vi "DidStop.vi"(8 "ErrorArray In":errorcluster[](array[cluster]), 10 "Init?":bool, 11 "NISTBus In":refnum<class "NISTBus.lvclass">) -> (0 "ErrorArray Out":errorcluster[](array[cluster]), 3 "NISTBus Out":refnum<class "NISTBus.lvclass">)   [LabVIEW 2014, in "Bus.lvlib"]
uses:
  Bus.lvlib
  NISTBus.lvclass
  Typedefs/clDidInit.ctl
  Typedefs/clUserEventType.ctl
  <userlib>/NIST/NISTErrorLib/NISTErrorLib.lvlib
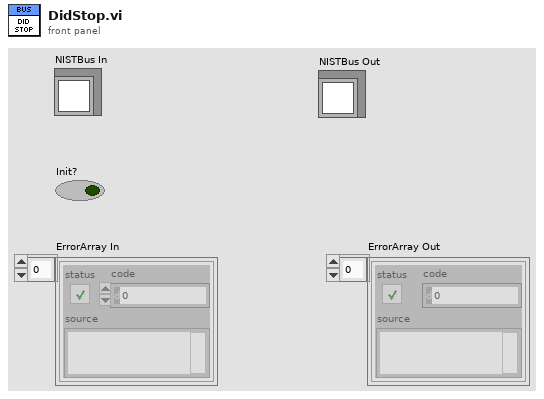
[diagram p1: front panel]
types:
  T1 = typedef "Bus.lvlib/clUserEventType.ctl" = cluster{"BusNumber":i8, "Data":variant}
  T2 = typedef "Bus.lvlib/clDidInit.ctl" = cluster{"NISTBus":refnum<vi>, "Init?":bool}
  T3 = typedef "Bus.lvlib/clBroadcastEvents.ctl" = cluster{"DidInit":refnum<user-event>, "DidStop":refnum<user-event>}
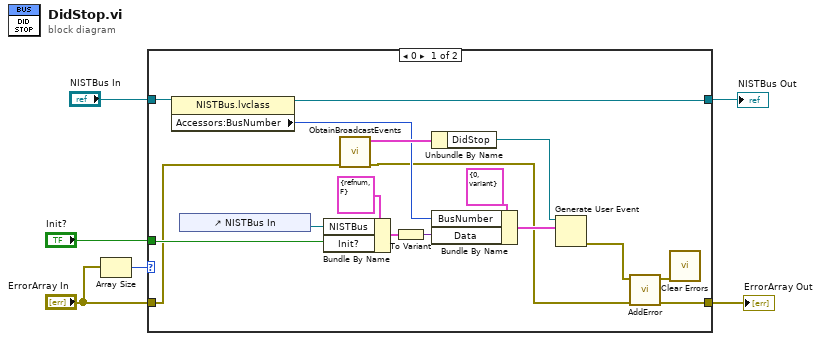
[diagram p0: block diagram]
diagram:
  n1 = Array Size(array="ErrorArray In") -> (size(s)=w6:i32)
  n2 = case shown="0" w6 {
    tunnel: "ErrorArray In" -> [w18 w24]
    tunnel: "Init?" -> [w19 _]
    tunnel: [w22 w25] -> w2
    tunnel: "NISTBus In" -> [w23 w25]
    tunnel: [w9 w24] -> w1
    frame 0 {
      n3 = property class="NISTBus.lvclass"(reference=w23) -> (reference out=w22:refnum<class "NISTBus.lvclass">, "Accessors:BusNumber"=w13:u8)  [unwired: 1 in, 1 out]
      n4 = control-ref of="NISTBus In"() -> (w20:refnum<vi>)
      n5 = Bundle By Name(cluster=T2 {"NISTBus"=refnum, "Init?"=FALSE} ("clNISTBusDidInit"), "NISTBus"=w20, "Init?"=w19) -> (w14:T2)
      n6 = call "ObtainBroadcastEvents.vi"("ErrorArray In"=w18) -> ("ErrorArray Out"=w7:errorcluster[], "NISTBusBroadcast"=w17:T3)  [unwired: 9 in]
      n7 = To Variant(anything=w14) -> (Variant=w15:variant)
      n8 = Unbundle By Name(w17) -> ("DidStop"=w11:refnum<user-event>)
      n9 = Bundle By Name(cluster=T1 {"BusNumber"=0, "Data"=variant} ("clEventType"), "BusNumber"=w13, "Data"=w15) -> (w12:T1)
      n10 = Generate User Event(user event=w11, event data cluster=w12) -> (error out=w8:errorcluster)  [unwired: 2 in, 1 out]
      n11 = call <userlib>:"AddError.vi"("ErrorArray"=w7, "error in (no error)"=w8) -> ("ErrorArray"=w9:errorcluster[], "error out"=w10:errorcluster)  [unwired: 8 in]
      n12 = call <vilib>:"Clear Errors.vi"("error in (no error)"=w10) -> ()  [unwired: 5 in, 2 out]
    }
    frame 1, Default {
    }
  }
  "NISTBus Out" <- w2
  "ErrorArray Out" <- w1
